vi "BigIntAdd.vi"(1 "b":cluster{"Boolean":bool, "Array":u64[]}, 2 "a":cluster{"Boolean":bool, "Array":u64[]}) -> (0 "a + b":cluster{"Boolean":bool, "Array":u64[]})   [LabVIEW 2023]
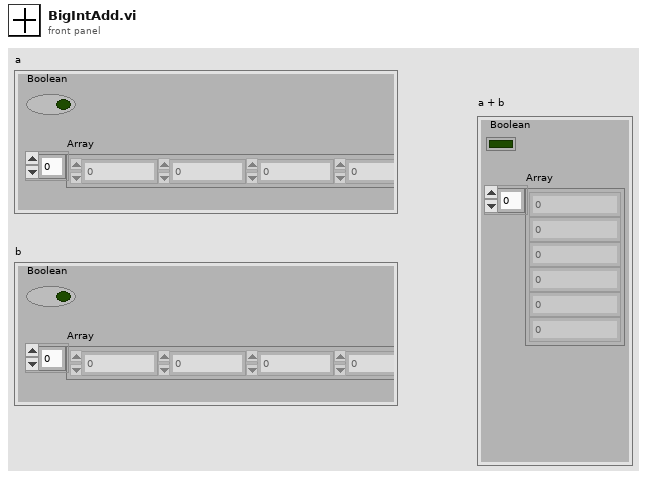
[diagram p1: front panel]
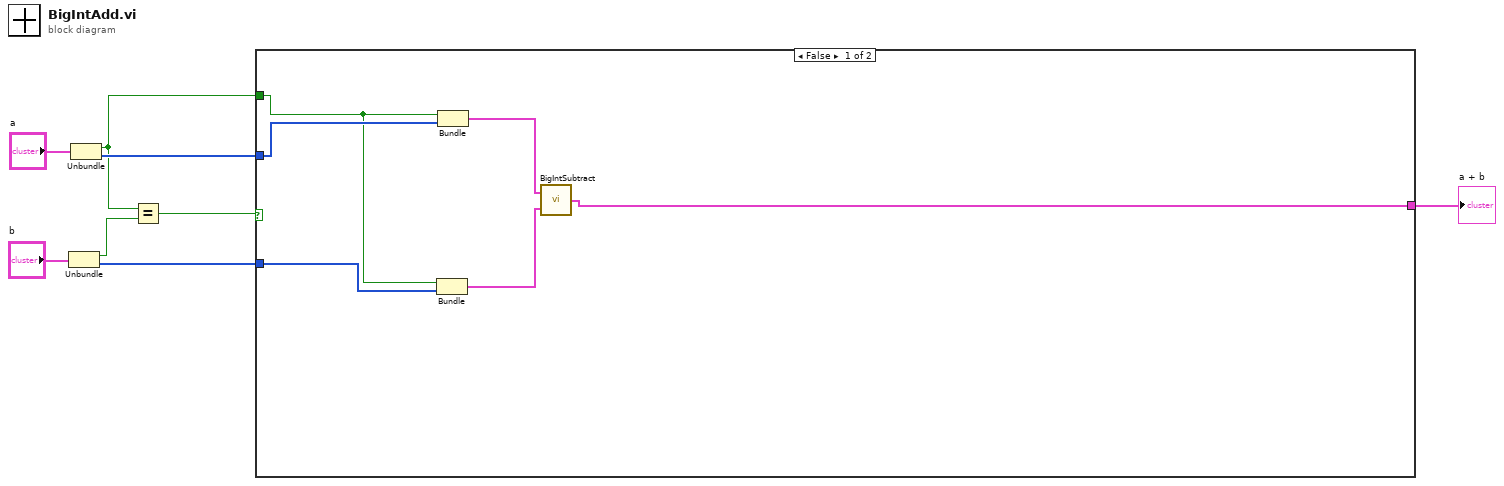
[diagram p0: block diagram]
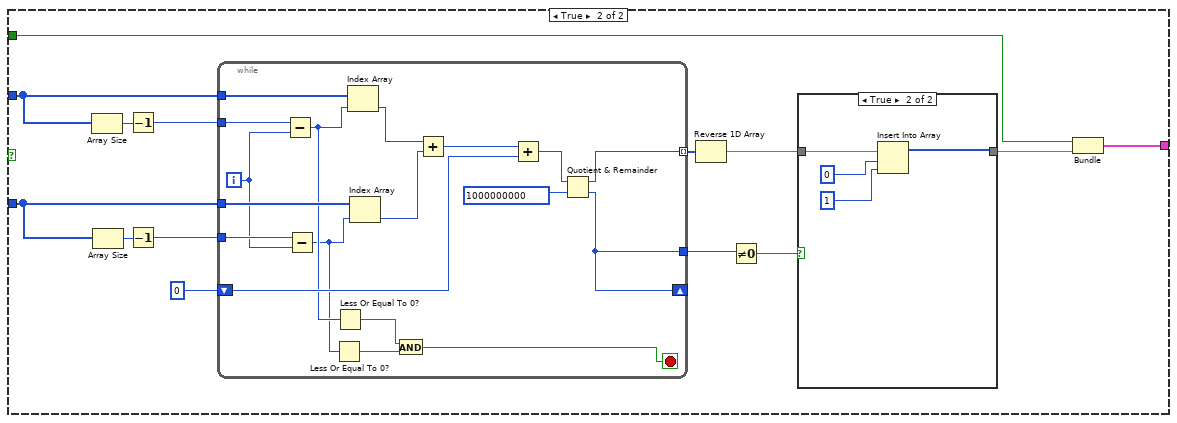
[diagram p2: hidden frame]
diagram:
  n1 = Unbundle("b") -> ("Boolean"=w1:bool, "Array"=w4:u64[])
  n2 = Unbundle("a") -> ("Boolean"=w3:bool, "Array"=w5:u64[])
  n3 = Equal?(x=w3, y=w1) -> (x = y?=w6:bool)
  n4 = case shown="False" w6 {
    tunnel: w5 -> [w14 w28]
    tunnel: w4 -> [w12 w27]
    tunnel: w3 -> [w13 w17]
    tunnel: [w9 w16] -> w2
    frame False {
      n5 = Bundle("Boolean"=w13, "Array"=w12) -> (w10:cluster{"Boolean":bool, "Array":u64[]})  [unwired: 1 in]
      n6 = Bundle("Boolean"=w13, "Array"=w14) -> (w11:cluster{"Boolean":bool, "Array":u64[]})  [unwired: 1 in]
      n7 = call "BigIntSubtract.vi"("b"=w10, "a"=w11) -> ("a - b"=w9:cluster{"Boolean":bool, "Array":u64[]})
    }
    frame True {
      n8 = Array Size(array=w28) -> (size(s)=w26:i32)
      n9 = Array Size(array=w27) -> (size(s)=w25:i32)
      n10 = Decrement(x=w26) -> (x-1=w24:i32)
      n11 = Decrement(x=w25) -> (x-1=w23:i32)
      n12 = while {
        tunnel: w28 -> [w51]
        tunnel: w27 -> [w49]
        tunnel: w24 -> [w50]
        tunnel: w23 -> [w48]
        shift-right: [w35] -> _
        shift-left: 0 -> [w45]
        tunnel: [w34] -> w20 mode=indexing
        tunnel: [w35] -> w21
        i -> [w43]
        stop <- w38 stop-if-true
        n13 = Subtract(x=w50, y=w43) -> (x-y=w42:i32)
        n14 = Subtract(x=w48, y=w43) -> (x-y=w41:i32)
        n15 = Less Or Equal To 0?(x=w41) -> (x <= 0?=w39:bool)
        n16 = Less Or Equal To 0?(x=w42) -> (x <= 0?=w40:bool)
        n17 = Index Array(array=w51, index=w42) -> (element=w47:u64)
        n18 = Index Array(array=w49, index=w41) -> (element=w46:u64)
        n19 = And(x=w40, y=w39) -> (x .and. y?=w38:bool)
        n20 = Add(x=w47, y=w46) -> (x+y=w44:u64)
        n21 = Add(x=w44, y=w45) -> (x+y=w37:u64)
        n22 = Quotient & Remainder(x=w37, y=1000000000) -> (x-y*floor(x/y)=w34:u64, floor(x/y)=w35:u64)
      }
      n23 = Reverse 1D Array(array=w20) -> (reversed array=w15:u64[])
      n24 = Not Equal To 0?(x=w21) -> (x != 0?=w19:bool)
      n25 = case shown="True" w19 {
        tunnel: w15 -> [w29 w33]
        tunnel: [w29 w30] -> w18
        frame False {
        }
        frame True {
          n26 = Insert Into Array(array=w33, index=0, new element=u64 1) -> (w30:u64[])
        }
      }
      n27 = Bundle("Boolean"=w17, w18) -> (w16:cluster{"Boolean":bool, u64[]})  [unwired: 1 in]
    }
  }
  "a + b" <- w2
